vi "Crosspoint_y.vi"(0 "Discharge X channels?":bool=TRUE, 1 "Y Channel Ground":string="y1", 2 "Array":string[](array[combo])=["NC", "NC", "NC", "NC", "NC", "NC", "NC", "NC"], 3 "Discharge Y Channels?":bool=TRUE, 4 "X Channel Ground":string="x12") -> ()   [LabVIEW 2016, in "pickering.lvclass"]
uses:
  pickering.lvclass
panel:
  in  "IVI Option String":string="Simulate=0,RangeCheck=1,QueryInstrStatus=0,Cache=1,DriverSetup=Model:40-726-511;"
  in  "VISA Resource Name":string="PXI9::13::INSTR"
  # "y1"
  # "y2"
  # "y3"
  # "y4"
  # "y5"
  # "y6"
  # "y7"
  # "y8"
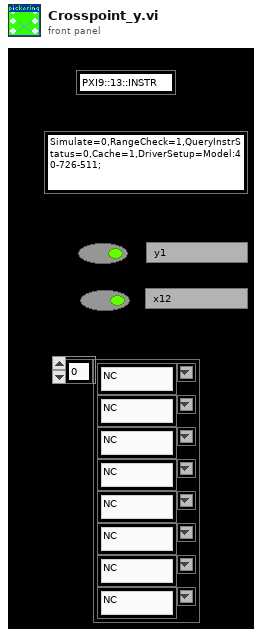
[diagram p1: front panel]
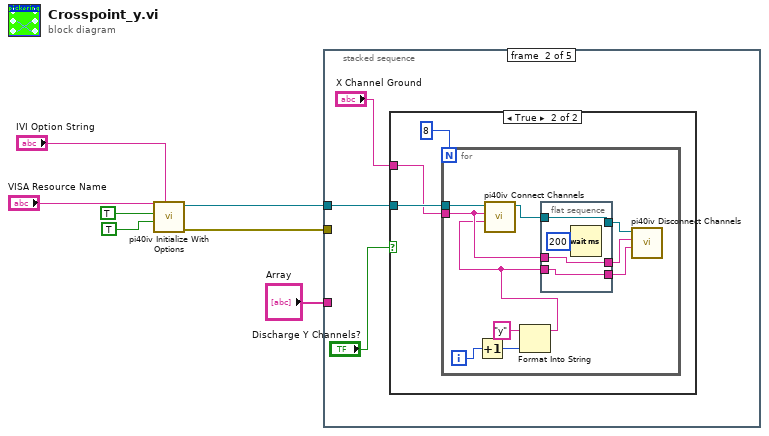
[diagram p0: block diagram]
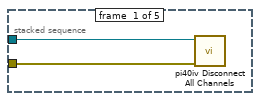
[diagram p2: hidden frame]
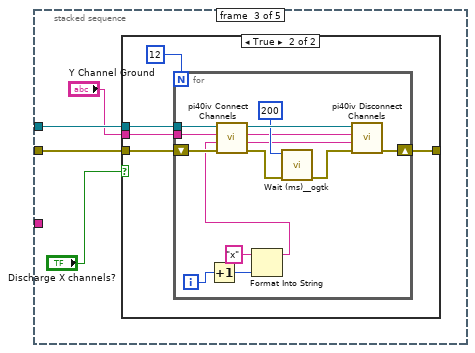
[diagram p4: hidden frame]
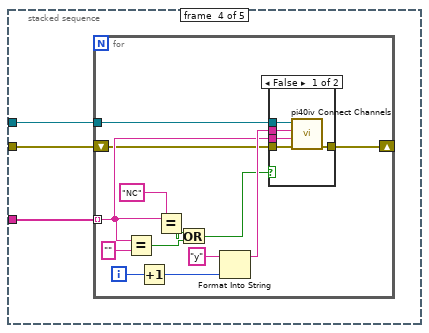
[diagram p6: hidden frame]
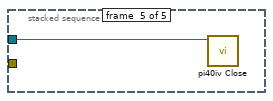
[diagram p8: hidden frame]
diagram:
  n1 = call <instrlib>:"pi40iv Initialize With Options.vi"("option string"="IVI Option String", "reset device"=TRUE, "id query"=TRUE, "resource name"="VISA Resource Name") -> ("error out"=w2:errorcluster, "instrument handle out"=w3:refnum<k15>)  [unwired: 6 in]
  n2 = stacked-sequence {
    tunnel: w3 -> [w9 w10 w33 w54 w74]
    tunnel: w2 -> [w8 _ w30 w52 _]
    tunnel: "Array" -> [_ _ _ w53 _]
    frame #0 {
      n3 = call <instrlib>:"pi40iv Disconnect All Channels.vi"("error in (no error)"=w8, "instrument handle"=w9) -> ()  [unwired: 8 in, 2 out]
    }
    frame #1 {
      n4 = case shown="True" "Discharge Y Channels?" {
        tunnel: w10 -> [_ w15]
        tunnel: "X Channel Ground" -> [_ w14]
        frame False {
        }
        frame True {
          n5 = for {
            N: 8 -> [_]
            tunnel: w15 -> [w25]
            tunnel: w14 -> [w22]
            i -> [w18]
            n6 = Increment(x=w18) -> (x+1=w16:i32)
            n7 = Format Into String(initial string="y", w16) -> (resulting string=w17:string)  [unwired: 2 in, 1 out]
            n8 = call <instrlib>:"pi40iv Connect Channels.vi"("channel 2"=w17, "channel 1"=w22, "instrument handle"=w25) -> ("instrument handle out"=w24:refnum<k15>)  [unwired: 7 in, 1 out]
            n9 = flat-sequence {
              tunnel: w24 -> [w29]
              tunnel: [w29] -> w23
              tunnel: w22 -> [w27]
              tunnel: [w27] -> w21
              tunnel: w17 -> [w26]
              tunnel: [w26] -> w20
              frame #0 {
                n10 = Wait (ms)(milliseconds to wait=u32 200) -> ()  [unwired: 1 out]
              }
            }
            n11 = call <instrlib>:"pi40iv Disconnect Channels.vi"("channel 2"=w20, "channel 1"=w21, "instrument handle"=w23) -> ()  [unwired: 7 in, 2 out]
          }
        }
      }
    }
    frame #2 {
      n12 = case shown="True" "Discharge X channels?" {
        tunnel: w33 -> [_ w39]
        tunnel: "Y Channel Ground" -> [_ w38]
        tunnel: w30 -> [w34 w36]
        tunnel: [w34 w35] -> _
        frame False {
        }
        frame True {
          n13 = for {
            N: 12 -> [_]
            tunnel: w39 -> [w51]
            tunnel: w38 -> [w41]
            shift-right: [w42] -> w35
            shift-left: w36 -> [w46]
            i -> [w48]
            n14 = Increment(x=w48) -> (x+1=w47:i32)
            n15 = Format Into String(initial string="x", w47) -> (resulting string=w40:string)  [unwired: 2 in, 1 out]
            n16 = call <instrlib>:"pi40iv Connect Channels.vi"("error in (no error)"=w46, "channel 2"=w40, "channel 1"=w41, "instrument handle"=w51) -> ("error out"=w44:errorcluster, "instrument handle out"=w50:refnum<k15>)  [unwired: 6 in]
            n17 = call <userlib>:"Wait (ms)__ogtk.vi"("error in (no error)"=w44, "milliseconds to wait"=u32 200) -> ("error out"=w43:errorcluster)  [unwired: 8 in, 1 out]
            n18 = call <instrlib>:"pi40iv Disconnect Channels.vi"("error in (no error)"=w43, "channel 2"=w40, "channel 1"=w41, "instrument handle"=w50) -> ("error out"=w42:errorcluster)  [unwired: 6 in, 1 out]
          }
        }
      }
    }
    frame #3 {
      n19 = for {
        tunnel: w54 -> [w67]
        tunnel: w53 -> [w60] mode=indexing
        shift-right: [w56] -> _
        shift-left: w52 -> [w57]
        i -> [w66]
        n20 = Equal?(x=w60, y="") -> (x = y?=w59:bool)
        n21 = Increment(x=w66) -> (x+1=w64:i32)
        n22 = Equal?(x=w60, y="NC") -> (x = y?=w61:bool)
        n23 = Or(x=w61, y=w59) -> (x .or. y?=w55:bool)
        n24 = Format Into String(initial string="y" ("string"), w64) -> (resulting string=w63:string)  [unwired: 2 in, 1 out]
        n25 = case shown="False" w55 {
          tunnel: w67 -> [w72 _]
          tunnel: w63 -> [w70 _]
          tunnel: w60 -> [w71 _]
          tunnel: w57 -> [w69 w73]
          tunnel: [w68 w73] -> w56
          frame False {
            n26 = call <instrlib>:"pi40iv Connect Channels.vi"("error in (no error)"=w69, "channel 2"=w71, "channel 1"=w70, "instrument handle"=w72) -> ("error out"=w68:errorcluster)  [unwired: 6 in, 1 out]
          }
          frame True {
          }
        }
      }
    }
    frame #4 {
      n27 = call <instrlib>:"pi40iv Close.vi"("instrument handle"=w74) -> ()  [unwired: 10 in, 1 out]
    }
  }
